vi "PH_Strings.indicate Text.vi"(2 "String to show":string, 4 "Caption.Text":string, 5 "error in (no error)":errorcluster) -> (19 "error out":errorcluster)   [LabVIEW 2014, in "PH_Common.lvlib"]
doc: "This VI is forseen to show some text. If wanted, this text can be saved to harddisk."
uses:
  PH_Common.lvlib
panel:
  in  "Save":bool
  in  "Delete":bool
  out "Indicator":string caption="Klemmen and Tagnames of Instance: Test-PP-PU-Beckhoff"
  # "PCS"
  # "3.2"
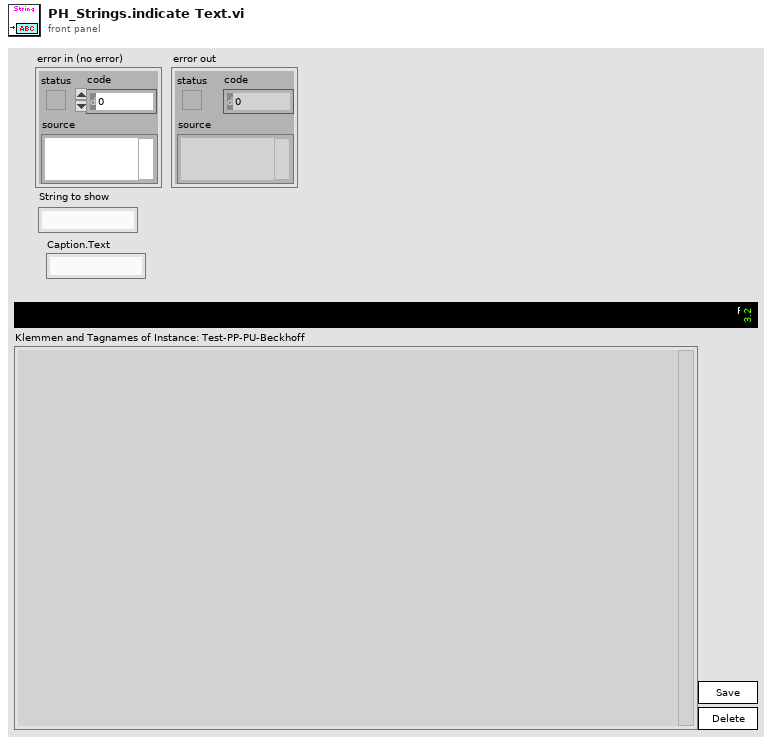
[diagram p1: front panel]
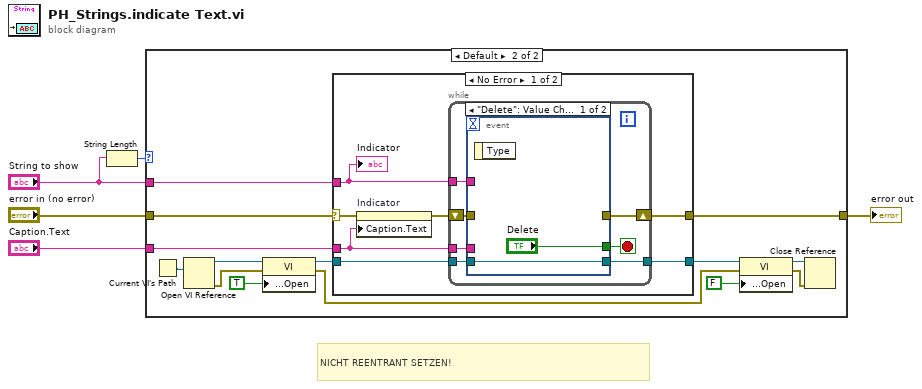
[diagram p0: block diagram]
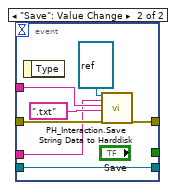
[diagram p3: hidden frame]
diagram:
  # "NICHT REENTRANT SETZEN!"
  n1 = String Length(string="String to show") -> (length=w1:i32)
  n2 = case shown="Default" w1 {
    tunnel: "String to show" -> [_ w20]
    tunnel: [w6 w19] -> w5
    tunnel: "error in (no error)" -> [w6 w8]
    tunnel: "Caption.Text" -> [_ w7]
    frame 0 {
    }
    frame Default {
      n3 = Current VI's Path() -> (path=w18:path)
      n4 = Open VI Reference(vi path=w18) -> (vi reference=w17:refnum<vi>, error out=w11:errorcluster)  [unwired: 5 in]
      n5 = property class="VI"(reference=w17, error in=w11, "Front Panel Window:Open"=TRUE) -> (reference out=w15:refnum<vi>, error out=w10:errorcluster)
      n6 = case shown="No Error" w8 {
        selector: w8 -> [w24 w45]
        tunnel: w20 -> [w25 _]
        tunnel: [w22 w45] -> w19
        tunnel: w15 -> [w27 w44]
        tunnel: [w26 w44] -> w13
        tunnel: w7 -> [w21 _]
        frame No Error {
          n7 = property on="Indicator" class="Str"(error in=w24, "Caption.Text"=w21) -> (error out=w23:errorcluster)  [unwired: 1 in, 1 out]
          n8 = while {
            tunnel: w27 -> [w34]
            tunnel: [w33] -> w26
            tunnel: w25 -> [w32]
            tunnel: w21 -> [w29]
            shift-right: [w30] -> w22
            shift-left: w23 -> [w31]
            stop <- w28 stop-if-true
            n9 = event shown="[0] \"Delete\": Value Change" {
              selector: _ -> [_ _]
              dyn-events: _ -> [_ _]
              timeout: _ -> [_ _]
              tunnel: w32 -> [_ w42]
              tunnel: [w36 w43] -> w33
              tunnel: w34 -> [w36 w43]
              tunnel: w31 -> [_ w38]
              tunnel: [_ w39] -> w30
              tunnel: w29 -> [_ w37]
              tunnel: ["Delete" _] -> w28
              event "Delete": Value Change {
                n10 = event-data() -> ()  [unwired: 1 in, 1 out]
              }
              event "Save": Value Change {
                n11 = event-data() -> ()  [unwired: 1 in, 1 out]
                n12 = call "PH_Interaction.Save String Data to Harddisk.vi"("i ref in"=refnum<vi> refnum, "Explanation (for Example: Column 1: xxx, ...)"=w37, "Data (for example: Columns)"=w42, "file name extension"=".txt" ("file name extinction"), "error in (no error)"=w38) -> ("error out"=w39:errorcluster)  [unwired: 12 in, 2 out]
              }
            }
          }
          "Indicator" <- w25
        }
        frame Error {
        }
      }
      n13 = property class="VI"(reference=w13, error in=w10, "Front Panel Window:Open"=FALSE) -> (reference out=w12:refnum<vi>, error out=w9:errorcluster)
      n14 = Close Reference(reference=w12, error in (no error)=w9) -> ()  [unwired: 1 out]
    }
  }
  "error out" <- w5
